vi "HTTP HEADER Parse Content-Length.vi"(10 "HTTP HEADERS":string) -> (2 "Content-Length":i32)   [LabVIEW 2011]
uses:
  <vilib>/regexp/Match Regular Expression.xnode
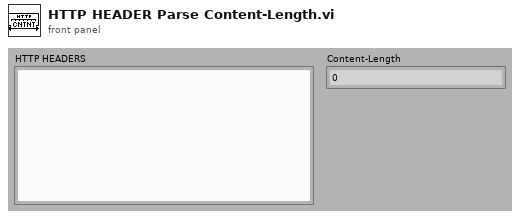
[diagram p1: front panel]
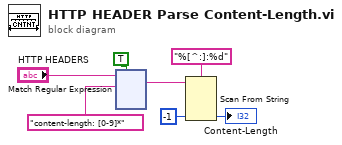
[diagram p0: block diagram]
diagram:
  n1 = xnode "Match Regular Expression"("input string"="HTTP HEADERS", "regular expression"="content-length: [0-9]*", "ignore case? (F)"=TRUE) -> ("whole match"=w5:string)  [unwired: 3 in, 4 out]
  n2 = Scan From String(format string="%[^:]:%d", input string=w5, default 2=-1 ("default value 2")) -> (output 2=→"Content-Length":i32)  [unwired: 4 in, 3 out]
